vi "set up acquisition parameters.vi"() -> ()   [LabVIEW 2014]
uses:
  Initilize Globals.vi
  lib/Andorlib/atmcd32d.lvlib
panel:
  out "Kinetics":dbl format="%#_13g"
  out "Accumulation":dbl format="%#_13g"
  out "Exposure":dbl format="%#_13g"
  in  "Acquisition Parametrs":T1
  out "error out":errorcluster
  in  "error in (no error)":errorcluster
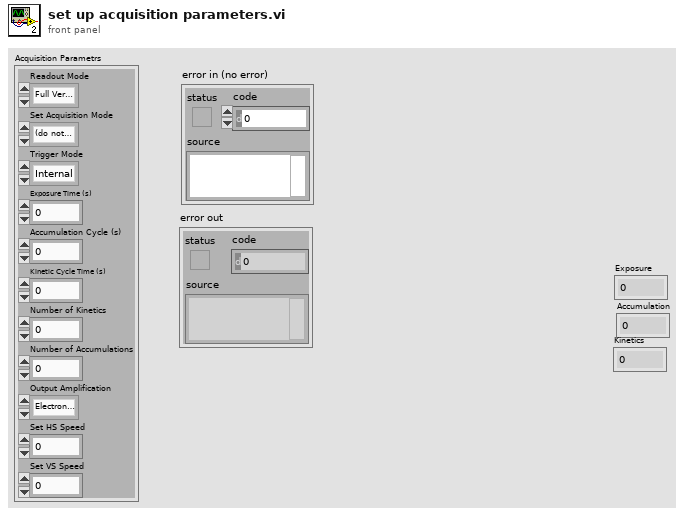
[diagram p1: front panel]
types:
  T1 = cluster{"Readout Mode":enum16{"Full Vertical Binning", "Multi-Track", "Random-Track", "Single-Track", "Image"}, "Set Acquisition Mode":enum16{"(do nothing)", "Single Scan", "Accumulate", "Kinetics", "Fast Kinetics", "Run till abort"}, "Trigger Mode":enum16{"Internal", "External"}, "Exposure Time (s)":dbl, "Accumulation Cycle (s)":dbl, "Kinetic Cycle Time (s)":dbl, "Number of Kinetics":i32, "Number of Accumulations":i32, "Output Amplification":enum16{"Electron Multiplication", "Extended NIR Mode"}, "Set HS Speed":i32, "Set VS Speed":i32}
  T2 = enum16{"Full Vertical Binning", "Multi-Track", "Random-Track", "Single-Track", "Image"}
  T3 = enum16{"(do nothing)", "Single Scan", "Accumulate", "Kinetics", "Fast Kinetics", "Run till abort"}
  T4 = enum16{"Electron Multiplication", "Extended NIR Mode"}
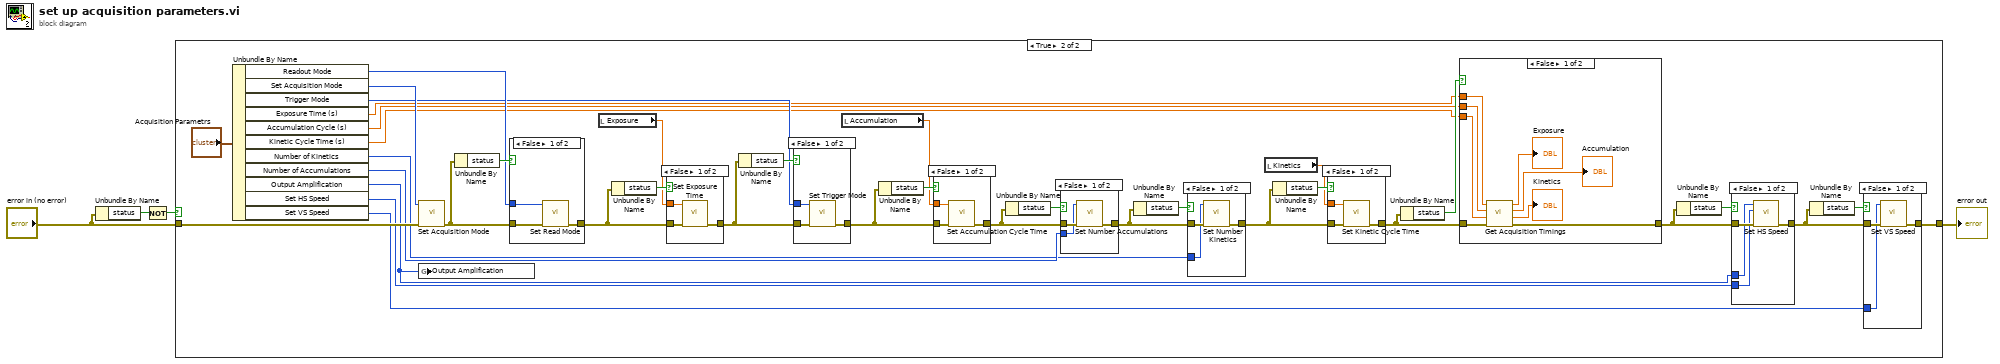
[diagram p0: block diagram]
diagram:
  n1 = Unbundle By Name("error in (no error)") -> ("status"=w4:bool)
  n2 = Not(x=w4) -> (.not. x?=w3:bool)
  n3 = case shown="True" w3 {
    tunnel: "error in (no error)" -> [w5 w42]
    tunnel: [w5 w25] -> w1
    frame False {
    }
    frame True {
      n4 = Unbundle By Name("Acquisition Parametrs") -> ("Readout Mode"=w18:T2, "Set Acquisition Mode"=w19:T3, "Trigger Mode"=w17:enum16{"Internal", "External"}, "Exposure Time (s)"=w10:dbl, "Accumulation Cycle (s)"=w11:dbl, "Kinetic Cycle Time (s)"=w9:dbl, "Number of Kinetics"=w15:i32, "Number of Accumulations"=w16:i32, "Output Amplification"=w12:T4, "Set HS Speed"=w14:i32, "Set VS Speed"=w13:i32)
      n5 = call "Set Acquisition Mode.vi"("error in (no error)"=w42, "mode"=w19) -> ("error out"=w23:errorcluster)  [unwired: 8 in, 1 out]
      n6 = global write "Initilize Globals.vi" "Output Amplification"(w12) -> ()
      n7 = Unbundle By Name(w23) -> ("status"=w24:bool)
      n8 = case shown="False" w24 {
        tunnel: w23 -> [w45 w46]
        tunnel: [w44 w46] -> w21
        tunnel: w18 -> [w43 _]
        frame False {
          n9 = call "Set Read Mode.vi"("error in (no error)"=w45, "mode"=w43) -> ("error out"=w44:errorcluster)  [unwired: 8 in, 1 out]
        }
        frame True {
        }
      }
      n10 = local read "Exposure"() -> (w8:dbl)
      n11 = Unbundle By Name(w21) -> ("status"=w22:bool)
      n12 = case shown="False" w22 {
        tunnel: w21 -> [w87 w88]
        tunnel: [w86 w88] -> w33
        tunnel: w8 -> [w85 _]
        frame False {
          n13 = call "Set Exposure Time.vi"("error in (no error)"=w87, "time"=w85) -> ("error out"=w86:errorcluster)  [unwired: 8 in, 1 out]
        }
        frame True {
        }
      }
      n14 = Unbundle By Name(w33) -> ("status"=w41:bool)
      n15 = case shown="False" w41 {
        tunnel: w33 -> [w83 w84]
        tunnel: [w82 w84] -> w32
        tunnel: w17 -> [w81 _]
        frame False {
          n16 = call "Set Trigger Mode.vi"("error in (no error)"=w83, "mode"=w81) -> ("error out"=w82:errorcluster)  [unwired: 8 in, 1 out]
        }
        frame True {
        }
      }
      n17 = local read "Accumulation"() -> (w7:dbl)
      n18 = Unbundle By Name(w32) -> ("status"=w40:bool)
      n19 = case shown="False" w40 {
        tunnel: w32 -> [w79 w80]
        tunnel: [w78 w80] -> w31
        tunnel: w7 -> [w77 _]
        frame False {
          n20 = call "Set Accumulation Cycle Time.vi"("error in (no error)"=w79, "time"=w77) -> ("error out"=w78:errorcluster)  [unwired: 8 in, 1 out]
        }
        frame True {
        }
      }
      n21 = Unbundle By Name(w31) -> ("status"=w39:bool)
      n22 = case shown="False" w39 {
        tunnel: w31 -> [w75 w76]
        tunnel: [w74 w76] -> w30
        tunnel: w16 -> [w73 _]
        frame False {
          n23 = call "Set Number Accumulations.vi"("error in (no error)"=w75, "number"=w73) -> ("error out"=w74:errorcluster)  [unwired: 8 in, 1 out]
        }
        frame True {
        }
      }
      n24 = Unbundle By Name(w30) -> ("status"=w38:bool)
      n25 = case shown="False" w38 {
        tunnel: w30 -> [w71 w72]
        tunnel: [w70 w72] -> w29
        tunnel: w15 -> [w69 _]
        frame False {
          n26 = call "Set Number Kinetics.vi"("error in (no error)"=w71, "number"=w69) -> ("error out"=w70:errorcluster)  [unwired: 8 in, 1 out]
        }
        frame True {
        }
      }
      n27 = local read "Kinetics"() -> (w6:dbl)
      n28 = Unbundle By Name(w29) -> ("status"=w37:bool)
      n29 = case shown="False" w37 {
        tunnel: w29 -> [w67 w68]
        tunnel: [w66 w68] -> w28
        tunnel: w6 -> [w65 _]
        frame False {
          n30 = call "Set Kinetic Cycle Time.vi"("error in (no error)"=w67, "time"=w65) -> ("error out"=w66:errorcluster)  [unwired: 8 in, 1 out]
        }
        frame True {
        }
      }
      n31 = Unbundle By Name(w28) -> ("status"=w36:bool)
      n32 = case shown="False" w36 {
        tunnel: w28 -> [w63 w64]
        tunnel: [w62 w64] -> w27
        tunnel: w11 -> [w61 _]
        tunnel: w10 -> [w60 _]
        tunnel: w9 -> [w59 _]
        frame False {
          n33 = call "Get Acquisition Timings.vi"("error in (no error)"=w63, "kinetic"=w59, "accumulate"=w61, "exposure"=w60) -> ("error out"=w62:errorcluster, "kinetic out"=→"Kinetics":sgl, "accumulate out"=→"Accumulation":sgl, "exposure out"=→"Exposure":sgl)  [unwired: 3 in, 1 out]
        }
        frame True {
        }
      }
      n34 = Unbundle By Name(w27) -> ("status"=w35:bool)
      n35 = case shown="False" w35 {
        tunnel: w27 -> [w54 w55]
        tunnel: [w53 w55] -> w26
        tunnel: w14 -> [w52 _]
        tunnel: w12 -> [w51 _]
        frame False {
          n36 = call "Set HS Speed.vi"("error in (no error)"=w54, "index"=w52, "typ"=w51) -> ("error out"=w53:errorcluster)  [unwired: 7 in, 1 out]
        }
        frame True {
        }
      }
      n37 = Unbundle By Name(w26) -> ("status"=w34:bool)
      n38 = case shown="False" w34 {
        tunnel: w26 -> [w49 w50]
        tunnel: [w48 w50] -> w25
        tunnel: w13 -> [w47 _]
        frame False {
          n39 = call "Set VS Speed.vi"("error in (no error)"=w49, "index"=w47) -> ("error out"=w48:errorcluster)  [unwired: 8 in, 1 out]
        }
        frame True {
        }
      }
    }
  }
  "error out" <- w1
